vi "cluster-head-to-file.vi"(0 "refnum in":refnum<file>, 3 "error in":errorcluster, 4 "cluster ref":refnum<vi>) -> (7 "refnum out":refnum<file>, 10 "error out":errorcluster)   [LabVIEW 2011]
panel:
  out "Label.Text":string
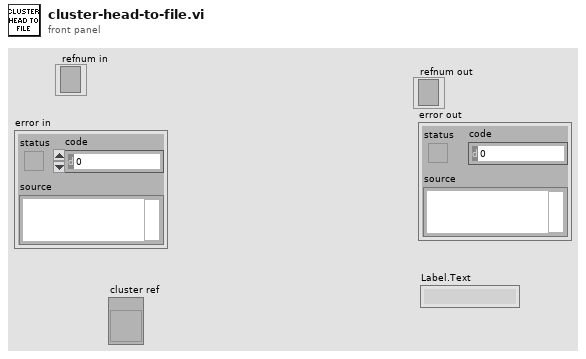
[diagram p1: front panel]
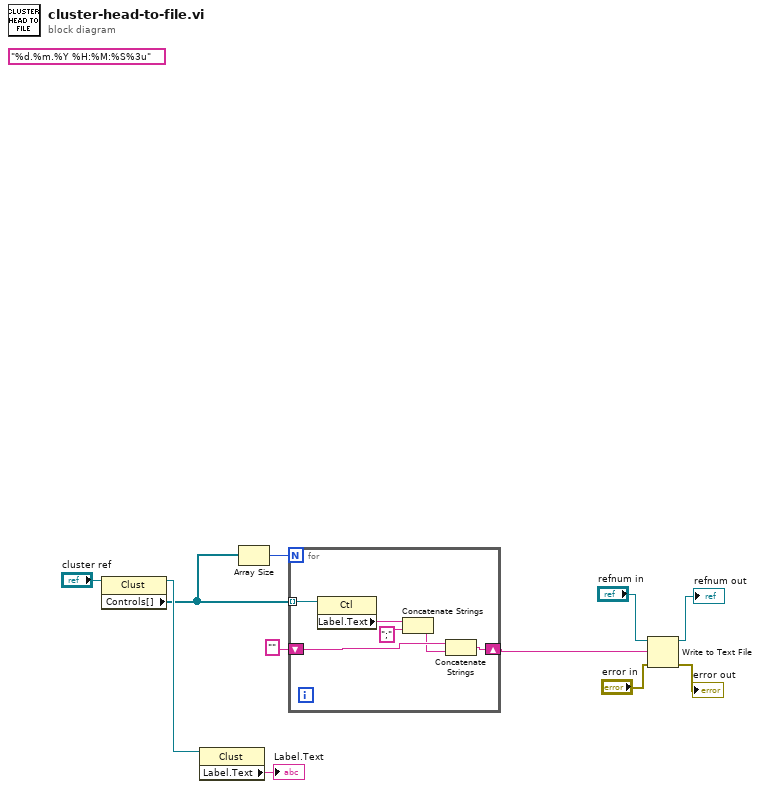
[diagram p0: block diagram]
diagram:
  (unwired) "%d.%m.%Y %H:%M:%S%3u" ("time format string (%c)")
  n1 = property class="Clust"(reference="cluster ref") -> (reference out=w7:refnum<vi>, "Controls[]"=w3:refnum<vi>[])  [unwired: 1 in, 1 out]
  n2 = property class="Clust"(reference=w7) -> ("Label.Text"=→"Label.Text":string)  [unwired: 1 in, 2 out]
  n3 = Array Size(array=w3) -> (size(s)=w2:i32)
  n4 = for {
    N: w2 -> [_]
    tunnel: w3 -> [w17] mode=indexing
    shift-right: [w14] -> w1
    shift-left: "" -> [w13]
    n5 = property class="Ctl"(reference=w17) -> ("Label.Text"=w15:string)  [unwired: 1 in, 2 out]
    n6 = Concatenate Strings(w15, ";") -> (w12:string)
    n7 = Concatenate Strings(w13, w12) -> (w14:string)
  }
  n8 = Write to Text File(file (use dialog)="refnum in", text=w1, error in="error in") -> (refnum out=→"refnum out":refnum<file>, error out=→"error out":errorcluster)  [unwired: 1 in, 1 out]
